vi "Get Temporary Image Directory+.vi"(8 "error in (no error)":errorcluster {"code" format="Error %.0f"}, 11 "VIDoc Printer - Confluence In":refnum<class "VIDoc Printer - Confluence.lvclass">) -> (0 "error out":errorcluster {"code" format="Error %.0f"}, 2 "Temporary Image Directory":path, 3 "VIDoc Printer - Confluence Out":refnum<class "VIDoc Printer - Confluence.lvclass">)   [LabVIEW 2023, in "VIDoc Printer - Confluence.lvlib" / "VIDoc Printer - Confluence.lvclass"]
uses:
  VIDoc Printer - Confluence.lvclass
  VIDoc Printer - Confluence.lvclass/VIDoc Printer - Confluence.ctl
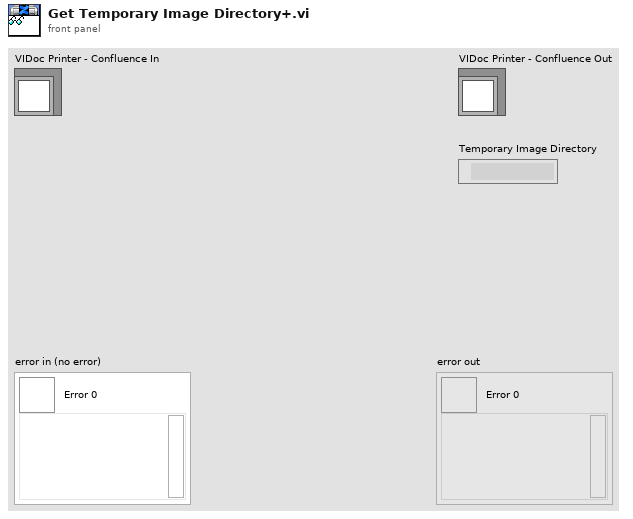
[diagram p1: front panel]
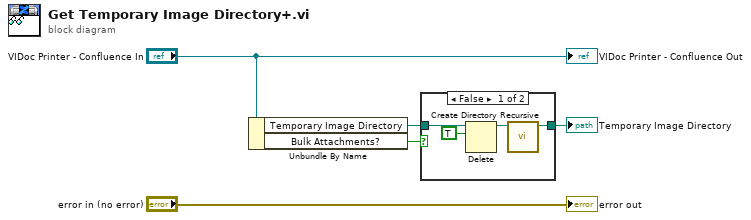
[diagram p0: block diagram]
diagram:
  n1 = Unbundle By Name("VIDoc Printer - Confluence In") -> ("Temporary Image Directory"=w3:path, "Bulk Attachments?"=w1:bool)
  n2 = case shown="False" w1 {
    tunnel: w3 -> [w7 w10]
    tunnel: [w6 w10] -> w2
    frame False {
      n3 = Delete(path (use dialog)=w7, entire hierarchy (F)=TRUE) -> (deleted path=w8:path)  [unwired: 3 in, 2 out]
      n4 = call <vilib>:"Create Directory Recursive.vi"("directory"=w8) -> ("directory copy"=w6:path)  [unwired: 4 in, 2 out]
    }
    frame True {
    }
  }
  "Temporary Image Directory" <- w2
  "error out" <- "error in (no error)"
  "VIDoc Printer - Confluence Out" <- "VIDoc Printer - Confluence In"
